vi "Get_Values.vi"(0 "reference in":refnum<class "AI.lvclass">) -> (6 "Data":T1 {"Stat Data"."scl mean 1Hz" format="%0.2f"; "Stat Data"."raw mean 1Hz" format="%0.2f"; "Stat Data"."scl mean" format="%0.2f"; "Stat Data"."raw mean" format="%0.2f"})   [LabVIEW 2019, in "AI.lvclass"]
uses:
  AI.lvclass
  TypeDef/AI_Data.ctl
  TypeDef/AI Statistics Data.ctl
  AI.lvclass/AI.ctl
  AnalogComparator_class/AnalogComparator.lvclass/AnalogComparator.ctl
  AnalogComparator_class/AnalogComparator.lvclass
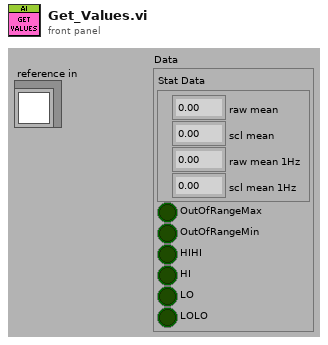
[diagram p1: front panel]
types:
  T1 = typedef "AI_Data.ctl" = cluster{"Stat Data":T2, "OutOfRangeMax":bool, "OutOfRangeMin":bool, "HIHI":bool, "HI":bool, "LO":bool, "LOLO":bool}
  T2 = typedef "AI Statistics Data.ctl" = cluster{"raw mean":dbl, "scl mean":dbl, "raw mean 1Hz":dbl, "scl mean 1Hz":dbl}
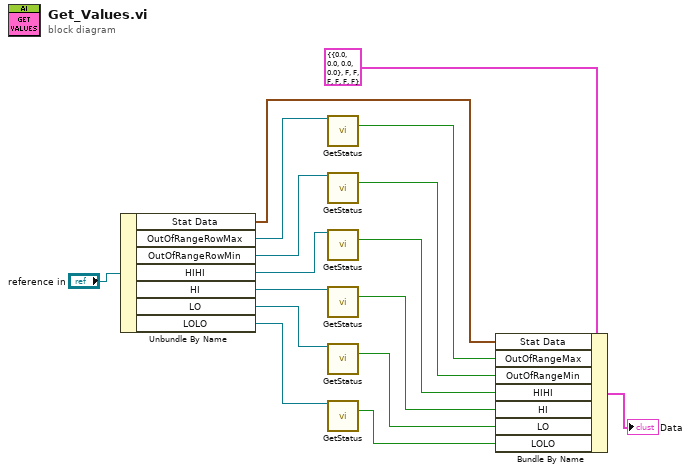
[diagram p0: block diagram]
diagram:
  n1 = Unbundle By Name("reference in") -> ("Stat Data"=w1:T2, "OutOfRangeRowMax"=w15:refnum<class "AnalogComparator.lvclass">, "OutOfRangeRowMin"=w13:refnum<class "AnalogComparator.lvclass">, "HIHI"=w12:refnum<class "AnalogComparator.lvclass">, "HI"=w11:refnum<class "AnalogComparator.lvclass">, "LO"=w10:refnum<class "AnalogComparator.lvclass">, "LOLO"=w9:refnum<class "AnalogComparator.lvclass">)
  n2 = call "GetStatus.vi"("class data in"=w15) -> ("Status"=w14:bool)  [unwired: 14 in]
  n3 = call "GetStatus.vi"("class data in"=w13) -> ("Status"=w8:bool)  [unwired: 14 in]
  n4 = call "GetStatus.vi"("class data in"=w12) -> ("Status"=w7:bool)  [unwired: 14 in]
  n5 = call "GetStatus.vi"("class data in"=w11) -> ("Status"=w6:bool)  [unwired: 14 in]
  n6 = call "GetStatus.vi"("class data in"=w10) -> ("Status"=w5:bool)  [unwired: 14 in]
  n7 = call "GetStatus.vi"("class data in"=w9) -> ("Status"=w4:bool)  [unwired: 14 in]
  n8 = Bundle By Name(cluster=T1 {"Stat Data"={"raw mean"=0.0, "scl mean"=0.0, "raw mean 1Hz"=0.0, "scl mean 1Hz"=0.0}, "OutOfRangeMax"=FALSE, "OutOfRangeMin"=FALSE, "HIHI"=FALSE, "HI"=FALSE, "LO"=FALSE, "LOLO"=FALSE} ("AI_Data"), "Stat Data"=w1, "OutOfRangeMax"=w14, "OutOfRangeMin"=w8, "HIHI"=w7, "HI"=w6, "LO"=w5, "LOLO"=w4) -> (→"Data":T1)
